vi "TempLogger_ReadyExit.vi"(0 "element":T1) -> (1 "Connected":bool, 2 "Exit System":bool)   [LabVIEW 2022 SP3]
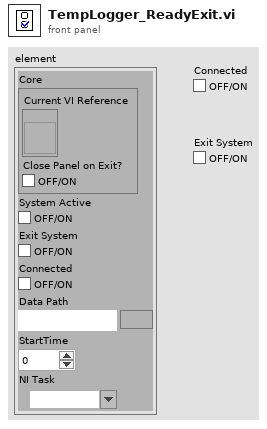
[diagram p1: front panel]
types:
  T1 = cluster{"Core":cluster{"Current VI Reference":refnum<vi>, "Close Panel on Exit?":bool}, "System Active":bool, "Exit System":bool, "Connected":bool, "Data Path":path, "StartTime":u32, "NI Task":refnum<k21>}
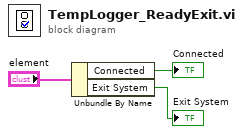
[diagram p0: block diagram]
diagram:
  n1 = Unbundle By Name("element") -> ("Connected"=→"Connected":bool, "Exit System"=→"Exit System":bool)
